vi "globalstop-example.vi"() -> ()   [LabVIEW 2017]
uses:
  user.lib/_NEVSTOP/GlobalStop/_gStop.vi
  user.lib/_NEVSTOP/GlobalStop/GSTOP.lvlib
panel:
  in  "stop Comp1\nIn Main Loop":bool
  in  "stop all":bool
  out "loop main":i32
  in  "stop Comp2":bool
  out "loop status":i32
  out "loop2":i32
  out "loop1":i32
  in  "stop Comp1":bool
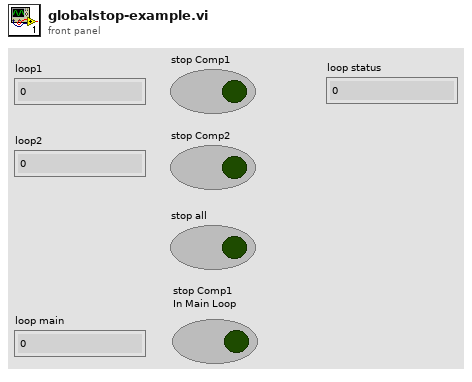
[diagram p1: front panel]
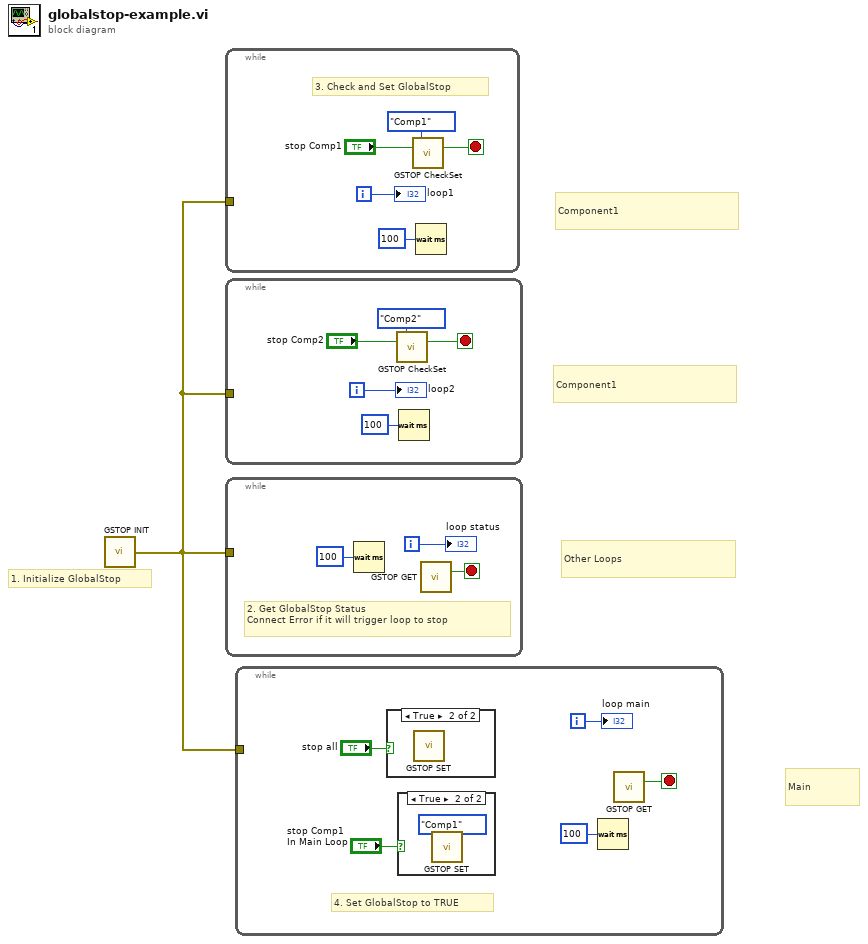
[diagram p0: block diagram]
diagram:
  # "1. Initialize GlobalStop"
  # "Main"
  # "Other Loops"
  # "Component1"
  # "Component1"
  n1 = call "GSTOP INIT.vi"() -> ("error out"=w1:errorcluster)  [unwired: 15 in]
  n2 = while {
    tunnel: w1 -> [_]
    i -> [w6]
    stop <- w4 stop-if-true
    # "3. Check and Set GlobalStop"
    n3 = call "GSTOP CheckSet.vi"("index(-1 for All)"=enum16{"Main", "Comp1", "Comp2"}."Comp1", "stop value"="stop Comp1") -> ("stop"=w4:bool)  [unwired: 12 in, 1 out]
    n4 = Wait (ms)(milliseconds to wait=100) -> ()  [unwired: 1 out]
    "loop1" <- w6
  }
  n5 = while {
    tunnel: w1 -> [_]
    i -> [w8]
    stop <- w10 stop-if-true
    n6 = call "GSTOP CheckSet.vi"("index(-1 for All)"=enum16{"Main", "Comp1", "Comp2"}."Comp2", "stop value"="stop Comp2") -> ("stop"=w10:bool)  [unwired: 12 in, 1 out]
    n7 = Wait (ms)(milliseconds to wait=100) -> ()  [unwired: 1 out]
    "loop2" <- w8
  }
  n8 = while {
    tunnel: w1 -> [_]
    i -> [w12]
    stop <- w13 stop-if-true
    # "2. Get GlobalStop Status\nConnect Error if it will trigger loop to stop"
    n9 = Wait (ms)(milliseconds to wait=100) -> ()  [unwired: 1 out]
    n10 = call "GSTOP GET.vi"() -> ("stop"=w13:bool)  [unwired: 14 in, 1 out]
    "loop status" <- w12
  }
  n11 = while {
    tunnel: w1 -> [_]
    i -> [w19]
    stop <- w16 stop-if-true
    # "4. Set GlobalStop to TRUE"
    n12 = case shown="True" "stop all" {
      frame False {
      }
      frame True {
        n13 = call "GSTOP SET.vi"() -> ()  [unwired: 15 in, 1 out]
      }
    }
    n14 = case shown="True" "stop Comp1\nIn Main Loop" {
      frame False {
      }
      frame True {
        n15 = call "GSTOP SET.vi"("index(-1 for All)"=enum16{"Main", "Comp1", "Comp2"}."Comp1") -> ()  [unwired: 14 in, 1 out]
      }
    }
    n16 = Wait (ms)(milliseconds to wait=100) -> ()  [unwired: 1 out]
    n17 = call "GSTOP GET.vi"() -> ("stop"=w16:bool)  [unwired: 14 in, 1 out]
    "loop main" <- w19
  }
